vi "ServiceHost.vi"(0 "error in":errorcluster, 2 "Topic":string="/junk", 3 "node":string) -> (1 "error out":errorcluster, 4 "Req":string)   [LabVIEW 2012]
doc: "Starts a service host on the RIO"
uses:
  <userlib>/ROSforLV/ROS/Code/Console/Servers/ServerSubs/TopicDef.ctl
  <userlib>/ROSforLV/ROS/Code/SubVIs/_ROSDirection.ctl
  <userlib>/ROSforLV/ROS/MessageParsing/std_msgs/subs/parse_string_scalar.vi
  <userlib>/ROSforLV/ROS/MessageBuilding/std_msgs/subs/stringScalar.vi
panel:
  out "msg out":string
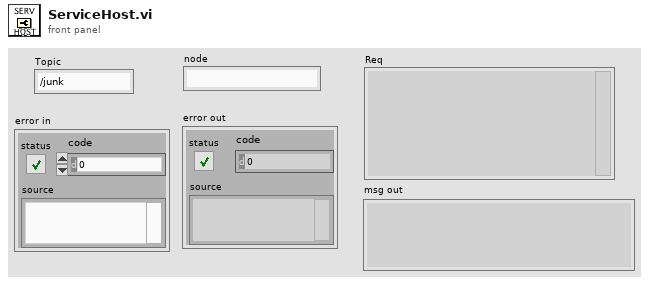
[diagram p1: front panel]
types:
  T1 = typedef "TopicDef.ctl" = cluster{"Topic":string, "Type":string, "Action":T2, "Update (ms)":u16, "queue size":u16}
  T2 = typedef "_ROSDirection.ctl" = enum16{"Node", "Publisher", "Subscriber", "ServiceClient", "ServiceProvider"}
  T3 = typedef "_ROSControl.ctl" = cluster{"topic port":u16, "Node":string, "topic":string, "type":string, "node port":u16, "error ":errorcluster, "Direction":T2, "Update (ms)":u16, "FIFO size":u16}
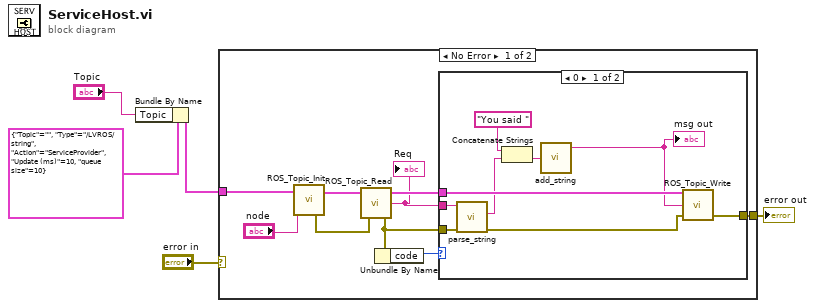
[diagram p0: block diagram]
diagram:
  n1 = Bundle By Name(cluster=T1 {"Topic"="", "Type"="/LVROS/string", "Action"=enum."ServiceProvider", "Update (ms)"=10, "queue size"=10} ("Definitions"), "Topic"="Topic") -> (w3:T1)
  n2 = case shown="No Error" "error in" {
    selector: "error in" -> [_ w25]
    tunnel: w3 -> [w13 _]
    tunnel: [w9 w25] -> w2
    frame No Error {
      n3 = call <userlib>:"ROS_Topic_Init.vi"("node"="node", "Definitions"=w13) -> ("error out"=w10:errorcluster, "ROS out"=w12:T3)
      n4 = call <userlib>:"ROS_Topic_Read.vi"("error in (no error)"=w10, "ROS in"=w12) -> ("error out"=w7:errorcluster, "Reply"=w8:string, "ROS out"=w11:T3)  [unwired: 1 in]
      "Req" <- w8
      n5 = Unbundle By Name(w7) -> ("code"=w6:i32)
      n6 = case shown="0" w6 {
        tunnel: w11 -> [w23 _]
        tunnel: [w19 w24] -> w9
        tunnel: w7 -> [w16 w24]
        tunnel: w8 -> [w15 _]
        frame 0 {
          n7 = call-poly <userlib>:"parse_string.vi"("error in"=w16, "msg in"=w15) -> ("error out"=w17:errorcluster, "string"=w22:string)  [unwired: 3 in, 1 out]
          n8 = Concatenate Strings("You said " ("string"), w22) -> (w21:string)
          n9 = call-poly <userlib>:"add_string.vi"("String"=w21) -> ("msg out"=w18:string)  [unwired: 4 in]
          "msg out" <- w18
          n10 = call <userlib>:"ROS_Topic_Write.vi"("error in (no error)"=w17, "Msg in"=w18, "ROS in"=w23) -> ("error out"=w19:errorcluster)  [unwired: 1 in, 1 out]
        }
        frame Default {
        }
      }
    }
    frame Error {
    }
  }
  "error out" <- w2
